vi "提取扭矩角度-4.vi"(11 "字符串":string="B1_011308090450260075.280040.000090.00A000002600000020009999AA ") -> (0 "角度值右":string, 1 "角度值左":string, 2 "扭矩值右":string, 3 "扭矩值左":string)   [LabVIEW 2013]
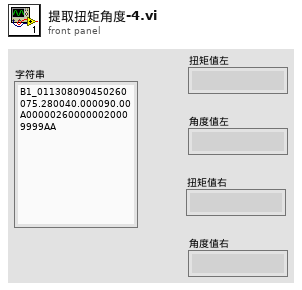
[diagram p1: front panel]
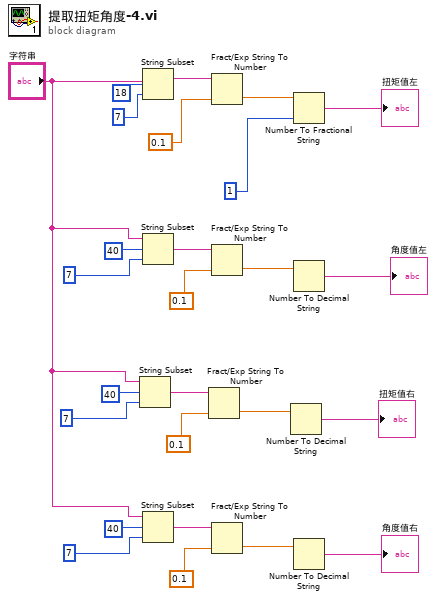
[diagram p0: block diagram]
diagram:
  n1 = String Subset(string="字符串", offset (0)=40 ("偏移量(0)"), length (rest)=7 ("长度（剩余）")) -> (substring=w11:string)
  n2 = String Subset(string="字符串", offset (0)=18 ("偏移量(0)"), length (rest)=7 ("长度（剩余）")) -> (substring=w19:string)
  n3 = String Subset(string="字符串", offset (0)=40 ("偏移量(0)"), length (rest)=7 ("长度（剩余）")) -> (substring=w22:string)
  n4 = String Subset(string="字符串", offset (0)=40 ("偏移量(0)"), length (rest)=7 ("长度（剩余）")) -> (substring=w5:string)
  n5 = Fract/Exp String To Number(string=w11, default (0 dbl)=0.1 ("默认(0 DBL)")) -> (number=w9:dbl)  [unwired: 2 in, 1 out]
  n6 = Fract/Exp String To Number(string=w19, default (0 dbl)=0.1 ("默认(0 DBL)")) -> (number=w18:dbl)  [unwired: 2 in, 1 out]
  n7 = Fract/Exp String To Number(string=w22, default (0 dbl)=0.1 ("默认(0 DBL)")) -> (number=w20:dbl)  [unwired: 2 in, 1 out]
  n8 = Fract/Exp String To Number(string=w5, default (0 dbl)=0.1 ("默认(0 DBL)")) -> (number=w3:dbl)  [unwired: 2 in, 1 out]
  n9 = Number To Decimal String(number=w9) -> (decimal integer string=→"扭矩值右":string)  [unwired: 1 in]
  n10 = Number To Fractional String(number=w18, precision (6)=i16 1 ("精度(6)")) -> (F-format string=→"扭矩值左":string)  [unwired: 2 in]
  n11 = Number To Decimal String(number=w20) -> (decimal integer string=→"角度值左":string)  [unwired: 1 in]
  n12 = Number To Decimal String(number=w3) -> (decimal integer string=→"角度值右":string)  [unwired: 1 in]
